vi "TextGetNumProperties.vi"(1 "Token":string, 2 "InputString":string) -> (0 "Numeric":i32)   [LabVIEW 2011]
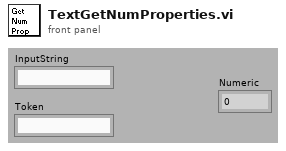
[diagram p1: front panel]
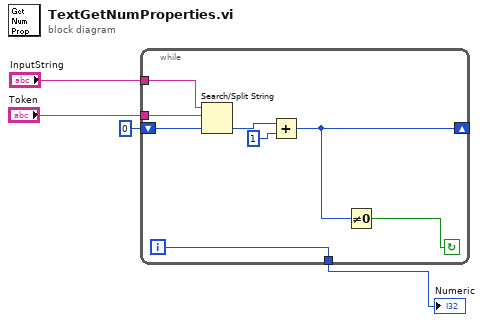
[diagram p0: block diagram]
diagram:
  n1 = while {
    shift-right: [w7] -> _
    shift-left: 0 -> [w10]
    tunnel: "Token" -> [w9]
    tunnel: "InputString" -> [w8]
    tunnel: [w5] -> w1
    i -> [w5]
    stop <- w6 continue-if-true
    n2 = Search/Split String(string=w8, search string/char (-)=w9, offset (0)=w10) -> (offset of match=w12:i32)  [unwired: 2 out]
    n3 = Add(x=w12, y=1) -> (x+y=w7:i32)
    n4 = Not Equal To 0?(x=w7) -> (x != 0?=w6:bool)
  }
  "Numeric" <- w1
